vi "Gaussian Filter(Pic1 LevelOther).vi"(0 "Height":u16, 1 "Width":u16, 2 "Rows":u16, 3 "Cols":u16, 5 "Memory in":refnum<k21>, 7 "Data in":fxp<+,12,12>, 9 "DV in":bool, 12 "DelayRowCount":i8) -> (6 "DV out":bool, 10 "Data Out":fxp<+,12,12>)   [LabVIEW 2016]
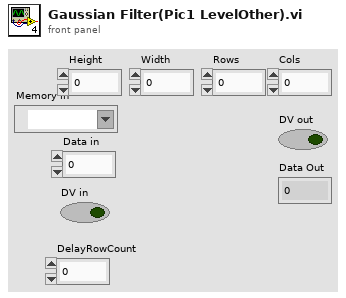
[diagram p1: front panel]
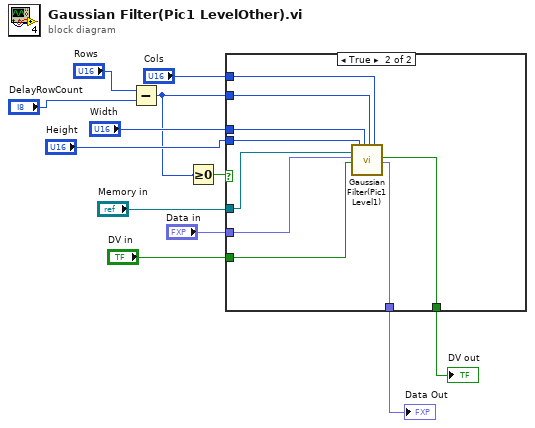
[diagram p0: block diagram]
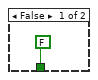
[diagram p2: hidden frame]
diagram:
  n1 = Subtract(x="Rows", y="DelayRowCount") -> (x-y=w1:u16)
  n2 = Greater Or Equal To 0?(x=w1) -> (x >= 0?=w2:bool)
  n3 = case shown="True" w2 {
    tunnel: "Cols" -> [_ w19]
    tunnel: w1 -> [_ w18]
    tunnel: "Width" -> [_ w17]
    tunnel: "Height" -> [_ w16]
    tunnel: "Data in" -> [_ w14]
    tunnel: "DV in" -> [_ w15]
    tunnel: "Memory in" -> [_ w20]
    tunnel: [FALSE ("DV out") w22] -> w12
    tunnel: [_ w21] -> w11
    frame False {
    }
    frame True {
      n4 = call "Gaussian Filter(Pic1 Level1).vi"("Memory In"=w20, "Data In"=w14, "DV In"=w15, "Height"=w16, "Width"=w17, "Rows"=w18, "Cols"=w19) -> ("DV out"=w22:bool, "Data Out"=w21:fxp<+,12,12>)  [unwired: 11 in]
    }
  }
  "DV out" <- w12
  "Data Out" <- w11
